vi "Log String.vi"(6 "String":string, 8 "error in (no error)":errorcluster, 11 "CSV File Sink in":refnum<class "CSV File Sink.lvclass">) -> (0 "error out":errorcluster, 3 "CSV File Sink out":refnum<class "CSV File Sink.lvclass">)   [LabVIEW 2016, in "Stream Log.lvlib" / "CSV File Sink.lvclass"]
doc: "--\nCopyright © 2017 Composed SystemsI All rights reserved.\n\nAuthor: Jon McBee <jon.mcbee@composed.io>\n\nThis library is provided \"AS IS\" ,WITHOUT WARRANTIES OR\nCONDITIONS OF ANY KIND, either express or implied.\n\nComposed Systems -- composed.io\n\nStream 0.0.1.1\nJon McBee - Composed Systems\nCopyright (c) 2017, Composed Systems"
uses:
  <userlib>/Composed Systems/Stream/Log/CSV File Sink/CSV File Sink.lvclass
  <userlib>/Composed Systems/Stream/Log/Text File Sink/Text File Sink.lvclass
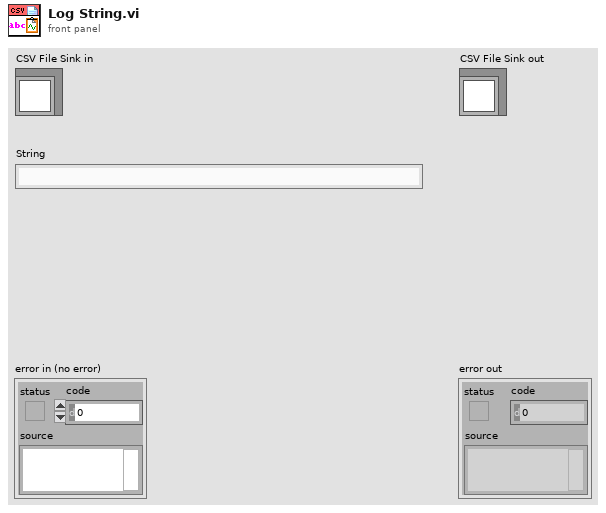
[diagram p1: front panel]
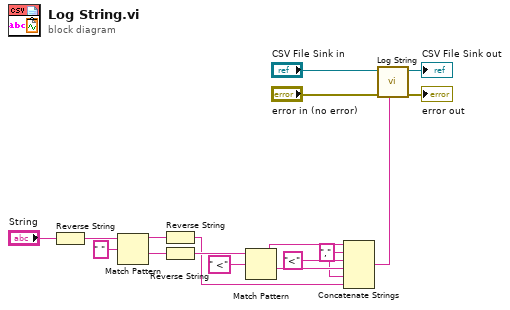
[diagram p0: block diagram]
diagram:
  w7 = "," ("string")
  n1 = Reverse String(1:"String") -> (0:w16:string)
  n2 = Match Pattern(string=w16, regular expression=" ") -> (before substring=w14:string, after substring=w13:string)  [unwired: 1 in, 2 out]
  n3 = Reverse String(1:w14) -> (0:w6:string)
  n4 = Reverse String(1:w13) -> (0:w12:string)
  n5 = Match Pattern(string=w12, regular expression=" <") -> (before substring=w8:string, after substring=w10:string)  [unwired: 1 in, 2 out]
  n6 = Concatenate Strings(w8, w7, "<" ("string"), w10, w7, w6) -> (w1:string)
  n7 = call-parent "Log String.vi"("String"=w1, "error in (no error)"="error in (no error)", "Text File Sink in"="CSV File Sink in") -> ("error out"=→"error out":errorcluster, "Text File Sink out"=→"CSV File Sink out":refnum<class "CSV File Sink.lvclass">)  [unwired: 7 in]
